vi "DisabledColor.vi"(1 "enabled":u32(colorbox)) -> (0 "disabled":u32(colorbox))   [LabVIEW 2014, in "PythonConverter_GUI.lvclass"]
uses:
  PythonConverter_GUI.lvclass
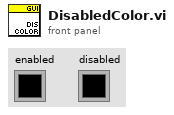
[diagram p1: front panel]
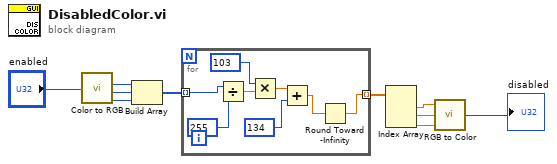
[diagram p0: block diagram]
diagram:
  n1 = call <vilib>:"Color to RGB.vi"("Color"="enabled") -> ("R"=w6:u8, "G"=w5:u8, "B"=w4:u8)  [unwired: 1 out]
  n2 = Build Array(w6, w5, w4) -> (w3:u8[])
  n3 = for {
    tunnel: w3 -> [w15] mode=indexing
    tunnel: [w11] -> w10 mode=indexing
    n4 = Divide(x=w15, y=u8 255 ("x")) -> (x/y=w14:dbl)
    n5 = Multiply(x=u8 103, y=w14) -> (x*y=w13:dbl)
    n6 = Add(x=w13, y=u8 134) -> (x+y=w12:dbl)
    n7 = Round Toward -Infinity(1:w12) -> (0:w11:dbl)
  }
  n8 = Index Array(array=w10) -> (element #1=w9:dbl, element #2=w8:dbl, element #3=w7:dbl)  [unwired: 3 in]
  n9 = call <vilib>:"RGB to Color.vi"("B"=w7, "G"=w8, "R"=w9) -> ("Color"=→"disabled":u32)
